vi "push-strlist.vi"(10 "string":string, 11 "target-list":string[](array[string])) -> (3 "output":string[](array[string]))   [LabVIEW 2019]
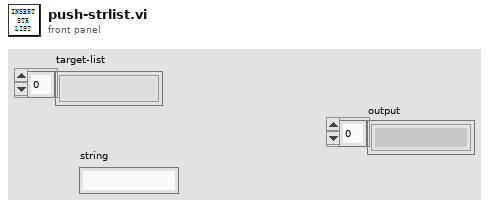
[diagram p1: front panel]
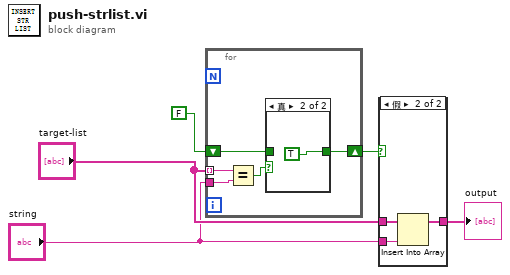
[diagram p0: block diagram]
diagram:
  n1 = for {
    tunnel: "target-list" -> [w10] mode=indexing
    tunnel: "string" -> [w9]
    shift-right: [w7] -> w3
    shift-left: FALSE -> [w6]
    n2 = Equal?(x=w10, y=w9) -> (x = y?=w8:bool)
    n3 = case shown="真" w8 {
      tunnel: [w11 TRUE] -> w7
      tunnel: w6 -> [w11 _]
      frame False {
      }
      frame True {
      }
    }
  }
  n4 = case shown="假" w3 {
    tunnel: "target-list" -> [w13 w16]
    tunnel: "string" -> [_ w15]
    tunnel: [w13 w14] -> w1
    frame True {
    }
    frame False {
      n5 = Insert Into Array(array=w16, new element=w15) -> (w14:string[])  [unwired: 1 in]
    }
  }
  "output" <- w1
